vi "Configure Power Measurement List Index Repetition.vi"(7 "Repetitions":i32[](array[numeric]), 8 "error in (no error)":errorcluster, 10 "Instance (1)":i32=1, 11 "VISA resource name":refnum<visa-resource-name>) -> (0 "error out":errorcluster, 3 "VISA resource name out":refnum<visa-resource-name>)   [LabVIEW 2015, in "Rohde&Schwarz CMXP GPRF.lvlib"]
doc: "Defines or queries the \"Index Repetion\" of all frequency/level steps.\n\nAttribute:\nRSCMXPGPRF_ATTR_POWER_MEASUREMENT_LIST_INDEX_REPETITION\n\nRemote-control command:\nCONFigure:GPRF:MEAS<i>:POWer:LIST:IREPetition:ALL"
uses:
  <instrlib>/Rohde&Schwarz CMXP GPRF/Rohde&Schwarz CMXP GPRF.lvlib
  <instrlib>/Rohde&Schwarz CMXP GPRF/Private/rsidr_core.llb/rsidr_core.lvlib
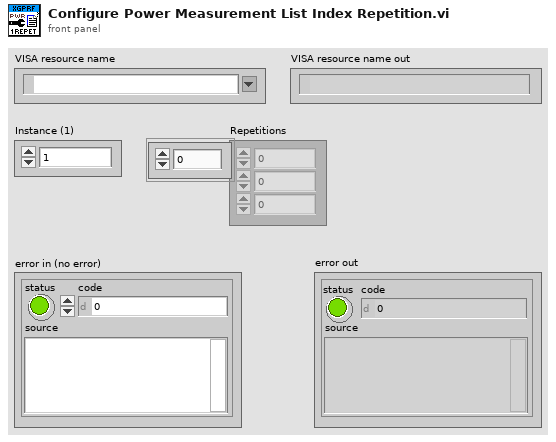
[diagram p1: front panel]
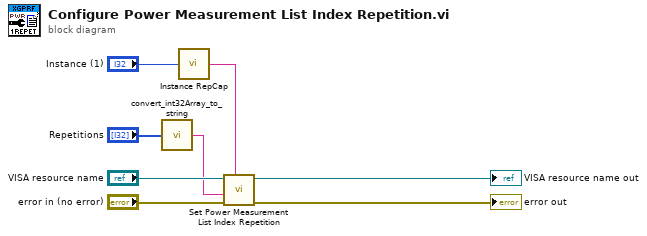
[diagram p0: block diagram]
diagram:
  n1 = call <instrlib>:"convert_int32Array_to_string.vi"("I32 array in"="Repetitions") -> ("string out"=w1:string)  [unwired: 4 in]
  n2 = call <instrlib>:"Instance RepCap.vi"("instance  in"="Instance (1)") -> ("instance out"=w5:string)
  n3 = call "Set Power Measurement List Index Repetition"("Repeated Capabilities"=w5, "error in (no error)"="error in (no error)", "Power Measurement List Index Repetition ()"=w1, "instrument handle"="VISA resource name") -> ("error out"=→"error out":errorcluster, "instrument handle out"=→"VISA resource name out":refnum<visa-resource-name>)  [unwired: 6 in]
